vi "ReadTDMS.vi"() -> ()   [LabVIEW 2013]
panel:
  out "通道名输出":string[](array[string])
  out "组名称输出":string
  out "波形图":waveform(dbl)[](graph)
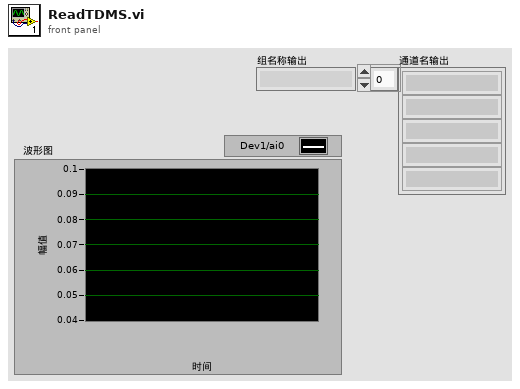
[diagram p1: front panel]
types:
  T1 = enum16{"open", "open or create", "create or replace", "create", "open (read-only)"}
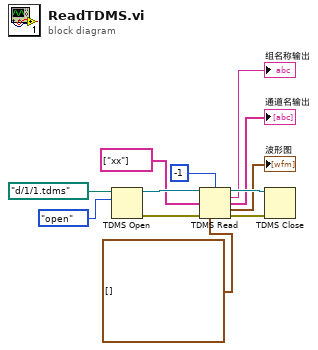
[diagram p0: block diagram]
diagram:
  n1 = TDMS Open(10:T1."open" ("操作(0:open)"), 11:path "d:/1/1.tdms" ("文件路径")) -> (0:w8:errorcluster, 3:w9:refnum<k34>)  [unwired: 5 in]
  n2 = TDMS Read(0:w9, 2:i64 -1 ("总数（-1:全部）"), 7:string[] ["xx"] ("通道名输入"), 11:w8, 12:waveform(dbl)[] [] ("数据")) -> (4:w10:refnum<k34>, 6:→"组名称输出":string, 8:→"通道名输出":string[], 10:→"波形图":waveform(dbl)[], 15:w7:errorcluster)  [unwired: 3 in, 1 out]
  n3 = TDMS Close(8:w7, 11:w10) -> ()  [unwired: 2 out]
